vi "CRYFlatten Messages.vi"(11 "Messages":T1={"Name"="Default", "Type"=0, "Command Msg"="<Enter message or command here>", "Flags"=0, "Dialog?"=FALSE, "Numeric?"=FALSE, "Wait?"=FALSE, "Pause [ms]"=0, "pattern"=0, "Address"="", "Operation"=0, "bytes"=0, "Line selected"=0, "RS232 Func"=0, "Serial Ctrl lines"=0, "Interf #"=0, "GPIB func"=0, "GPIB cmd"=0, "GPIB rem en"=FALSE, "GPIB term"=0, "Curves generated"=[], "Units"={"unit"="", "dB ref"=0.0, "axis"=0, "data"=0, "Common dB ref."=1}, "Axis"=0, "Default Value"=0.0, "Message Tilte"="", "Port #"=0, "Print Unit"="", "Text Format"={"Size"=0, "Plain"=FALSE, "Bold"=FALSE, "Italic"=FALSE, "Underline"=FALSE, "Strikethrough"=FALSE, "Color"=0, "Font"=""}, "Help"="", "Tab Value"=enum."Setting", "pattern 2"=0, "Line selected 2"=0, "H_Bits"=[], "G_Bits"=[]} {"pattern 2" format="%.0b"; "Units"."Common dB ref." items=["dB", "dBSPL", "dBPa", "dBV", "dBm", "dBu", "dBFS"]; "Units"."dB ref" format="%.2p"; "pattern" format="%.0b"; "Flags" items=["Pass", "Fail"]}) -> (3 "Flatten Messages String":string)   [LabVIEW 2013]
uses:
  Typedef Control/CRYMessages Cluster.ctl
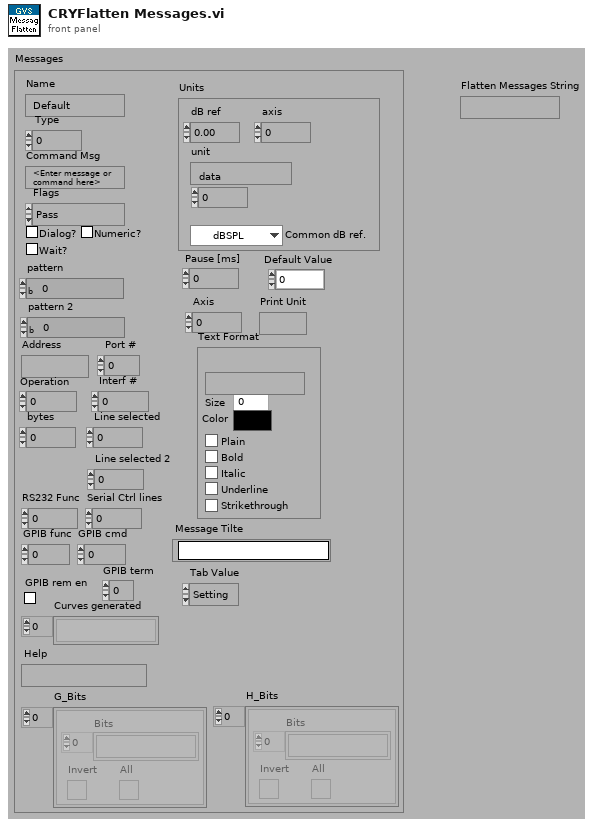
[diagram p1: front panel]
types:
  T1 = typedef "CRYMessages Cluster.ctl" = cluster{"Name":string, "Type":u16, "Command Msg":string, "Flags":u16, "Dialog?":bool, "Numeric?":bool, "Wait?":bool, "Pause [ms]":i32, "pattern":u32, "Address":string, "Operation":i32, "bytes":i32, "Line selected":u32, "RS232 Func":u16, "Serial Ctrl lines":u16, "Interf #":u8, "GPIB func":u16, "GPIB cmd":u16, "GPIB rem en":bool, "GPIB term":i32, "Curves generated":string[], "Units":cluster{"unit":string, "dB ref":dbl, "axis":u16, "data":u16, "Common dB ref.":u16}, "Axis":u16, "Default Value":dbl, "Message Tilte":string, "Port #":i32, "Print Unit":string, "Text Format":cluster{"Size":u32, "Plain":bool, "Bold":bool, "Italic":bool, "Underline":bool, "Strikethrough":bool, "Color":u32, "Font":string}, "Help":string, "Tab Value":enum32{"Setting", "Help"}, "pattern 2":u32, "Line selected 2":u32, "H_Bits":cluster{"Bits":string[], "Invert":bool, "All":bool}[], "G_Bits":cluster{"Bits":string[], "Invert":bool, "All":bool}[]}
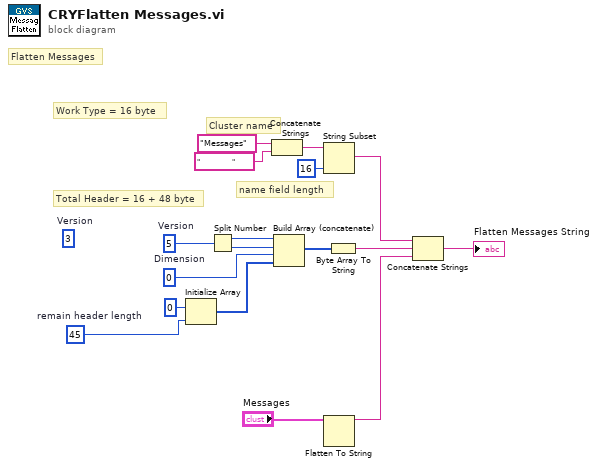
[diagram p0: block diagram]
diagram:
  (unwired) u16 3  # Version
  w9 = u16 5  # Version
  w12 = u8 0  # Dimension
  w8 = 45  # remain header length
  # "name field length"
  # "Cluster name"
  # "Flatten Messages"
  # "Work Type = 16 byte"
  # "Total Header = 16 + 48 byte"
  n1 = Initialize Array(u8 0 ("element"), w8) -> (w14:u8[])
  n2 = Split Number(x=w9) -> (hi(x)=w10:u8, lo(x)=w11:u8)
  n3 = Concatenate Strings("Messages" ("string"), "                " ("string")) -> (w5:string)
  n4 = Build Array (concatenate)(w10, w11, w12, w14) -> (w13:u8[])
  n5 = String Subset(string=w5, length (rest)=16 ("length (rest)")) -> (substring=w17:string)  [unwired: 1 out]
  n6 = Flatten To String(anything="Messages") -> (data string=w15:string)  [unwired: 1 in, 4 out]
  n7 = Byte Array To String(unsigned byte array=w13) -> (string=w16:string)
  n8 = Concatenate Strings(w17, w16, w15) -> (→"Flatten Messages String":string)
